vi "Configuration reader.vi"(0 "refnum":T1, 7 "error in (no error)":errorcluster) -> (1 "Velocity":dbl, 2 "Exposure":dbl(slide)=99.80425000000001 min=0.06241666666666667 max=99.80425000000001 step=0.06241666666666667 scale=0.06241666666666667..99.80425000000001 scale format="%#.3g", 3 "X offset":i32=693 step=1, 4 "Y travel":dbl min=0.0 max=5.0 step=0.0001, 5 "X travel":dbl min=0.0 max=50.0 step=0.0001, 8 "Y offset":i32=406 step=1, 9 "Acceleration":dbl, 10 "Pixelclock":i32(slide)=24 min=5 max=40 step=1 scale=5.0..40.0, 11 "Framerate":dbl(slide)=10.002522802986672 min=0.47411700449083627 max=15.001275108384213 step=0.014032998230481021 scale=0.47411700449083627..15.001275108384213 scale format="%#.3g", 12 "Width (px)":i32=240, 13 "Speed (µm/s)":i32=1000, 14 "XPS_Address":string, 15 "Axis 1 group":i32, 16 "Precision (%)":dbl=1.0 min=1.0 max=100.0 step=1.0 format="%#_3g", 17 "Pixel size":dbl=12.19 step=0.01, 18 "Axis 2 inverted?":bool, 19 "Axis 1 inverted?":bool, 20 "Heigth (px)":i32=240, 21 "Laser Com Delay":i32, 23 "Height  step \ndivider":i32=2, 24 "VISA Laser port":string, 25 "Axis 2 group":i32, 27 "error out":errorcluster)   [LabVIEW 2016]
uses:
  <vilib>/Utility/config.llb/Config Data RefNum.ctl
  <vilib>/Utility/config.llb/Read Key (I32).vi
  <vilib>/Utility/config.llb/Read Key (Double).vi
  <vilib>/Utility/config.llb/Read Key (String).vi
  <vilib>/Utility/config.llb/Read Key (Boolean).vi
  <vilib>/Utility/config.llb/NI_LVConfig.lvlib
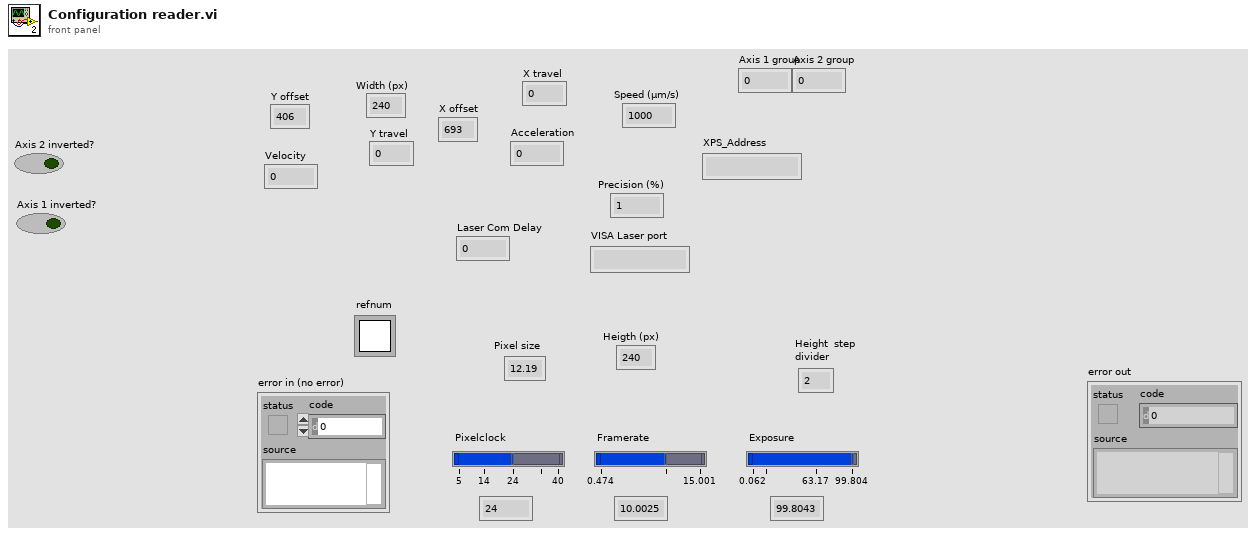
[diagram p1: front panel]
types:
  T1 = typedef "NI_LVConfig.lvlib/Config Data RefNum.ctl" = refnum<k1>
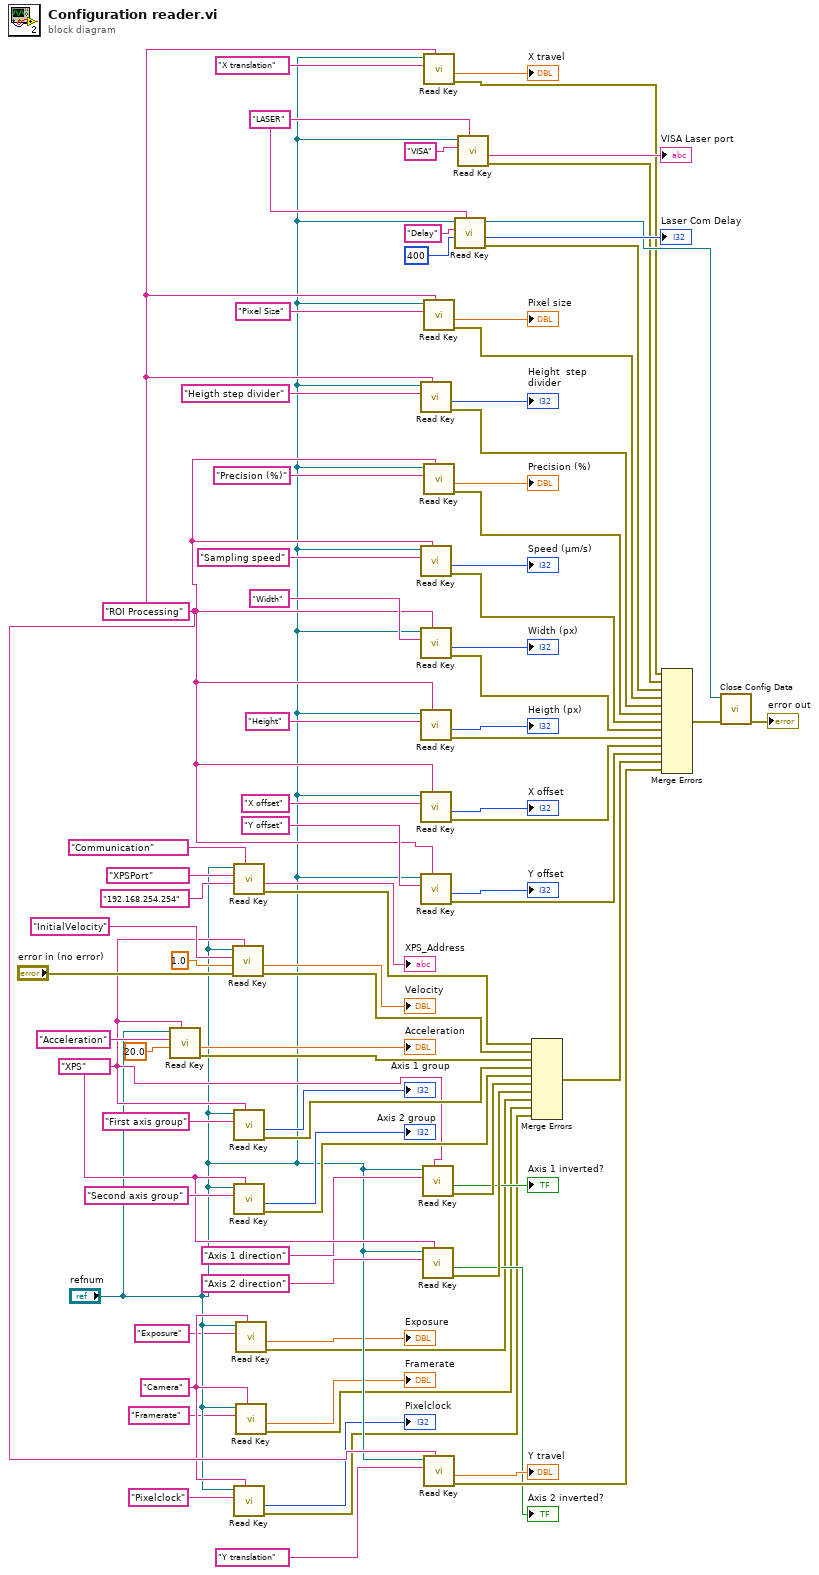
[diagram p0: block diagram]
diagram:
  w11 = "Camera" ("section")
  w34 = "LASER" ("section")
  w50 = "ROI Processing" ("section")
  w14 = "XPS" ("section")
  n1 = call-poly <vilib>:"Read Key.vi"("section"=w14, "default value"=20.0, "key"="Acceleration", "refnum"="refnum") -> ("error out"=w51:errorcluster, "value"=→"Acceleration":dbl)  [unwired: 4 in, 2 out]
  n2 = call-poly <vilib>:"Read Key.vi"("section"=w14, "error in (no error)"="error in (no error)", "default value"=1.0, "key"="InitialVelocity", "refnum"="refnum") -> ("error out"=w52:errorcluster, "value"=→"Velocity":dbl)  [unwired: 3 in, 2 out]
  n3 = call-poly <vilib>:"Read Key.vi"("section"="Communication", "default value"="192.168.254.254", "key"="XPSPort", "refnum"="refnum") -> ("error out"=w53:errorcluster, "value"=→"XPS_Address":string)  [unwired: 4 in, 2 out]
  n4 = call-poly <vilib>:"Read Key.vi"("section"=w14, "key"="First axis group", "refnum"="refnum") -> ("error out"=w19:errorcluster, "value"=→"Axis 1 group":i32)  [unwired: 5 in, 2 out]
  n5 = call-poly <vilib>:"Read Key.vi"("section"=w14, "key"="Second axis group", "refnum"="refnum") -> ("error out"=w22:errorcluster, "value"=→"Axis 2 group":i32)  [unwired: 5 in, 2 out]
  n6 = call-poly <vilib>:"Read Key.vi"("section"=w11, "key"="Pixelclock", "refnum"="refnum") -> ("error out"=w3:errorcluster, "value"=→"Pixelclock":i32)  [unwired: 5 in, 2 out]
  n7 = call-poly <vilib>:"Read Key.vi"("section"=w11, "key"="Exposure", "refnum"="refnum") -> ("error out"=w1:errorcluster, "value"=→"Exposure":dbl)  [unwired: 5 in, 2 out]
  n8 = call-poly <vilib>:"Read Key.vi"("section"=w11, "key"="Framerate", "refnum"="refnum") -> ("error out"=w2:errorcluster, "value"=→"Framerate":dbl)  [unwired: 5 in, 2 out]
  n9 = call-poly <vilib>:"Read Key.vi"("section"=w50, "key"="Heigth step divider", "refnum"="refnum") -> ("error out"=w62:errorcluster, "value"=→"Height  step \ndivider":i32)  [unwired: 5 in, 2 out]
  n10 = call-poly <vilib>:"Read Key.vi"("section"=w50, "key"="Sampling speed", "refnum"="refnum") -> ("error out"=w60:errorcluster, "value"=→"Speed (µm/s)":i32)  [unwired: 5 in, 2 out]
  n11 = call-poly <vilib>:"Read Key.vi"("section"=w50, "key"="Width", "refnum"="refnum") -> ("error out"=w59:errorcluster, "value"=→"Width (px)":i32)  [unwired: 5 in, 2 out]
  n12 = call-poly <vilib>:"Read Key.vi"("section"=w50, "key"="Height", "refnum"="refnum") -> ("error out"=w58:errorcluster, "value"=→"Heigth (px)":i32)  [unwired: 5 in, 2 out]
  n13 = call-poly <vilib>:"Read Key.vi"("section"=w50, "key"="X offset", "refnum"="refnum") -> ("error out"=w57:errorcluster, "value"=→"X offset":i32)  [unwired: 5 in, 2 out]
  n14 = call-poly <vilib>:"Read Key.vi"("section"=w50, "key"="Y offset", "refnum"="refnum") -> ("error out"=w56:errorcluster, "value"=→"Y offset":i32)  [unwired: 5 in, 2 out]
  n15 = call-poly <vilib>:"Read Key.vi"("section"=w14, "key"="Axis 1 direction", "refnum"="refnum") -> ("error out"=w17:errorcluster, "value"=→"Axis 1 inverted?":bool)  [unwired: 5 in, 2 out]
  n16 = call-poly <vilib>:"Read Key.vi"("section"=w14, "key"="Axis 2 direction", "refnum"="refnum") -> ("error out"=w18:errorcluster, "value"=→"Axis 2 inverted?":bool)  [unwired: 5 in, 2 out]
  n17 = call-poly <vilib>:"Read Key.vi"("section"=w50, "key"="X translation", "refnum"="refnum") -> ("error out"=w20:errorcluster, "value"=→"X travel":dbl)  [unwired: 5 in, 2 out]
  n18 = call-poly <vilib>:"Read Key.vi"("section"=w50, "key"="Pixel Size", "refnum"="refnum") -> ("error out"=w63:errorcluster, "value"=→"Pixel size":dbl)  [unwired: 5 in, 2 out]
  n19 = call-poly <vilib>:"Read Key.vi"("section"=w50, "key"="Precision (%)", "refnum"="refnum") -> ("error out"=w61:errorcluster, "value"=→"Precision (%)":dbl)  [unwired: 5 in, 2 out]
  n20 = call-poly <vilib>:"Read Key.vi"("section"=w50, "key"="Y translation", "refnum"="refnum") -> ("error out"=w21:errorcluster, "value"=→"Y travel":dbl)  [unwired: 5 in, 2 out]
  n21 = call-poly <vilib>:"Read Key.vi"("section"=w34, "default value"=400, "key"="Delay", "refnum"="refnum") -> ("error out"=w28:errorcluster, "value"=→"Laser Com Delay":i32, "refnum out"=w29:T1)  [unwired: 4 in, 1 out]
  n22 = call-poly <vilib>:"Read Key.vi"("section"=w34, "key"="VISA", "refnum"="refnum") -> ("error out"=w27:errorcluster, "value"=→"VISA Laser port":string)  [unwired: 5 in, 2 out]
  n23 = Merge Errors(w53, w52, w51, w19, w22, w17, w18, w1, w2, w3) -> (w54:errorcluster)
  n24 = Merge Errors(w20, w27, w28, w63, w62, w61, w60, w59, w58, w57, w56, w54, w21) -> (w55:errorcluster)
  n25 = call <vilib>:"Close Config Data.vi"("error in (no error)"=w55, "refnum"=w29) -> ("error out"=→"error out":errorcluster)  [unwired: 8 in, 1 out]
